vi "SetXL_AllCellValues.vi"(8 "error in (no error)":errorcluster, 10 "data":string[][](array[string]), 11 "Refnum Cluster Out in":T1) -> (0 "error out":errorcluster, 3 "Refnum Cluster Out out":T1)   [LabVIEW 2017, in "excel_configuration.lvlib"]
uses:
  excel_configuration.lvlib
  SetXL_CellValues_2D_String.vi
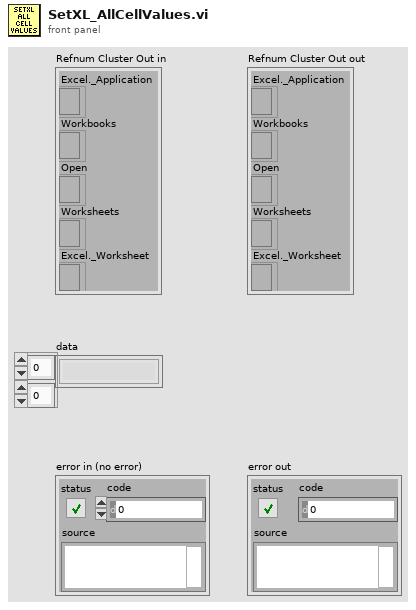
[diagram p1: front panel]
types:
  T1 = cluster{"Excel._Application":refnum<k7>, "Workbooks":refnum<k7>, "Open":refnum<k7>, "Worksheets":refnum<k7>, "Excel._Worksheet":refnum<k7>}
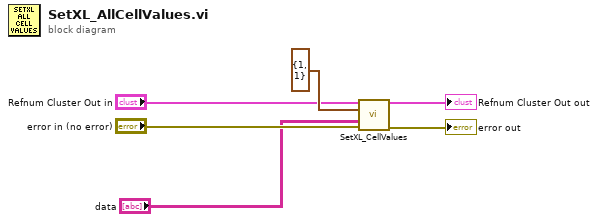
[diagram p0: block diagram]
diagram:
  n1 = call-poly "SetXL_CellValues.vi"("Refnum Cluster In"="Refnum Cluster Out in", "Start"=cluster{"Column":i32, "Row":i32} {"Column"=1, "Row"=1}, "data"="data", "error in"="error in (no error)") -> ("Refnum Cluster Out"=→"Refnum Cluster Out out":T1, "error out"=→"error out":errorcluster)  [unwired: 10 in]
